vi "XML Text Replace.vi"(9 "Text":string, 10 "Tag":string, 11 "XML in":string) -> (3 "XML out":string)   [LabVIEW 2021, in "BS120x Driver.lvlib" / "ENET_BS1200.lvclass"]
uses:
  ENET_BS1200.lvclass
panel:
  out "Original Text":string
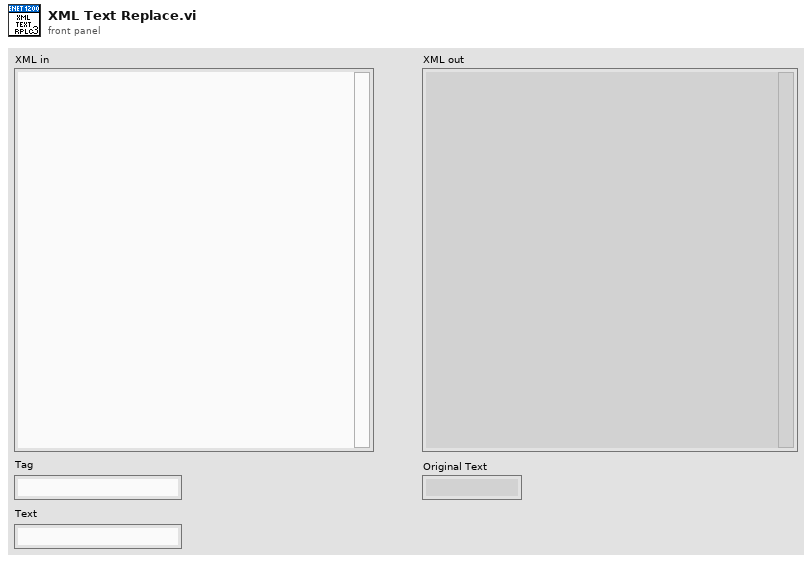
[diagram p1: front panel]
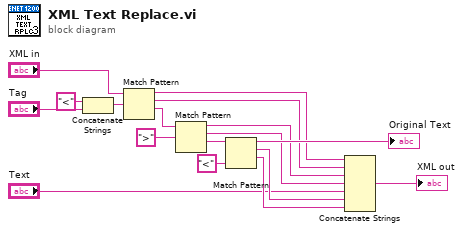
[diagram p0: block diagram]
diagram:
  n1 = Concatenate Strings("<" ("string"), "Tag") -> (w13:string)
  n2 = Match Pattern(string="XML in", regular expression=w13) -> (before substring=w3:string, match substring=w4:string, after substring=w17:string)  [unwired: 1 in, 1 out]
  n3 = Match Pattern(string=w17, regular expression=">") -> (before substring=w5:string, match substring=w6:string, after substring=w12:string)  [unwired: 1 in, 1 out]
  n4 = Match Pattern(string=w12, regular expression="<") -> (before substring=→"Original Text":string, match substring=w8:string, after substring=w9:string)  [unwired: 1 in, 1 out]
  n5 = Concatenate Strings(w3, w4, w5, w6, "Text", w8, w9) -> (→"XML out":string)
